vi "Set Switch Heating Time.vi"(1 "error in":T2, 2 "Switch Heating Time (sec)":dbl=15.0 min=5.0 max=120.0, 3 "Communications Config":T1={"GPIB address"=22, "GPIB bus"=0, "connection ID"=refnum, "IP"="192.168.2.200", "Active Comm Interface"=0, "Serial Port"="", "Programmer Type"=0} {"Programmer Type" items=["Model 430", "Model 420"]; "Active Comm Interface" items=["TCP/IP (Model 430 Only)", "RS232", "IEEE488"]}) -> (0 "error out":T2)   [LabVIEW 2018]
panel:
  in  "GPIB Address":cluster{"GPIB address":i16, "GPIB bus":i16}={"GPIB address"=22, "GPIB bus"=0}
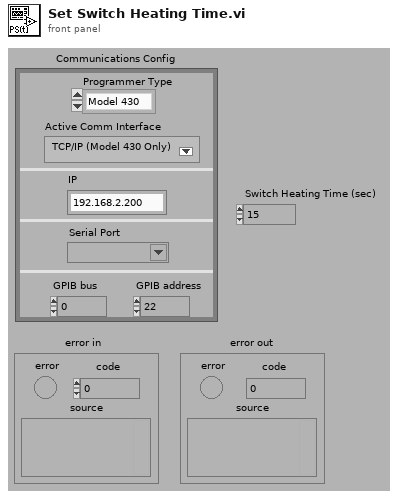
[diagram p1: front panel]
types:
  T1 = cluster{"GPIB address":i16, "GPIB bus":i16, "connection ID":refnum<k5>, "IP":string, "Active Comm Interface":u16, "Serial Port":refnum<visa-resource-name>, "Programmer Type":u16}
  T2 = cluster{"error":bool, "code":i32, "source":string}
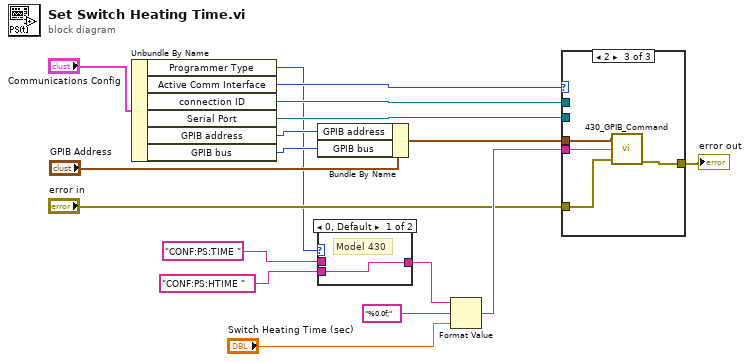
[diagram p0: block diagram]
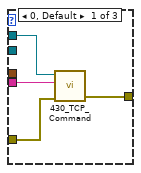
[diagram p3: hidden frame]
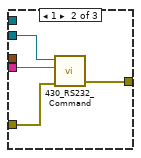
[diagram p4: hidden frame]
diagram:
  n1 = Unbundle By Name("Communications Config") -> ("Programmer Type"=w1:u16, "Active Comm Interface"=w4:u16, "connection ID"=w7:refnum<k5>, "Serial Port"=w6:refnum<visa-resource-name>, "GPIB address"=w9:i16, "GPIB bus"=w8:i16)
  n2 = Bundle By Name(cluster="GPIB Address", "GPIB address"=w9, "GPIB bus"=w8) -> (w3:cluster{"GPIB address":i16, "GPIB bus":i16})
  n3 = case shown="0, Default" w1 {
    tunnel: "CONF:PS:TIME " -> [_ w19]
    tunnel: "CONF:PS:HTIME " -> [w18 _]
    tunnel: [w18 w19] -> w10
    frame 0, Default {
      # "Model 430"
    }
    frame 1 {
      # "Model 420"
    }
  }
  n4 = Format Value(string ("")=w10, format string="%0.0f;", value (0)="Switch Heating Time (sec)") -> (output string=w15:string)
  n5 = case shown="2" w4 {
    tunnel: w15 -> [w21 w25 w31]
    tunnel: "error in" -> [w22 w26 w30]
    tunnel: [w23 w27 w29] -> w13
    tunnel: w7 -> [w20 _ _]
    tunnel: w6 -> [_ w24 _]
    tunnel: w3 -> [_ _ w28]
    frame 0, Default {
      n6 = call "430_TCP_Command.vi"("error in (no error)"=w22, "Command"=w21, "connection ID"=w20) -> ("error out"=w23:errorcluster)  [unwired: 1 in, 2 out]
    }
    frame 1 {
      n7 = call "430_RS232_Command.vi"("error in (no error)"=w26, "Command"=w25, "VISA resource name"=w24) -> ("error out"=w27:errorcluster)  [unwired: 1 in, 2 out]
    }
    frame 2 {
      n8 = call "430_GPIB_Command.vi"("GPIB (In)"=w28, "Input command"=w31, "error in"=w30) -> ("error out"=w29:T2)  [unwired: 3 out]
    }
  }
  "error out" <- w13
